vi "test_TCP_TCP Write.vi"(8 "error in (no error)":errorcluster, 11 "TestCase in":refnum<class "Ethernet Protocol Tests.lvclass">) -> (0 "error out":errorcluster, 3 "TestCase out":refnum<class "Ethernet Protocol Tests.lvclass">)   [LabVIEW 2019, in "Ethernet Protocol Tests.lvclass"]
uses:
  Ethernet Protocol Tests.lvclass
  ListenerVi/TCP/TCP.lvclass
  D:/GitRepository/niveristand-instrument-addon-classes/Source/Protocols/Tests/ListenerVi/Protocol Parent/Protocol Parent.lvclass
  ListenerVi/Listener.lvclass
  ListenerVi/ListenerClassControls/Operation Ctl.ctl
  ListenerVi/TCP/TCP.lvclass/TCP.ctl
  <vilib>/addons/_JKI Toolkits/VI Tester/TestCase.llb/TestCase.lvclass
  C:/Program Files (x86)/National Instruments/LabVIEW 2019/vi.lib/addons/_JKI Toolkits/VI Tester/TestCase.llb/TestCase.lvclass
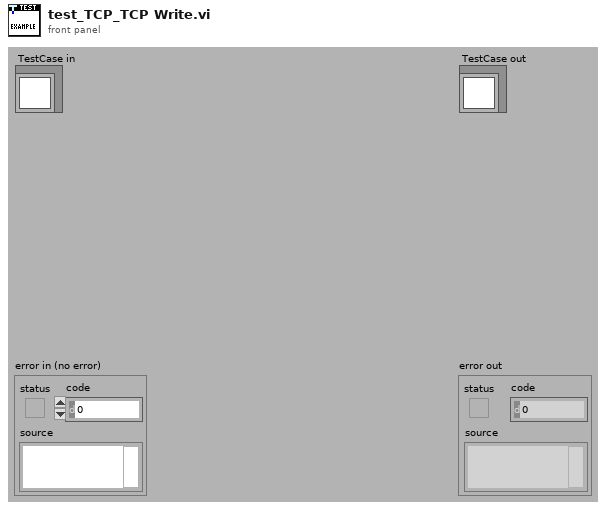
[diagram p1: front panel]
types:
  T1 = typedef "Operation Ctl.ctl" = enum16{"Read", "Write"}
  T2 = typedef "Listener.lvclass/TCP IP Data Structure.ctl" = cluster{"TCP|IP connection ID":refnum<k5>, "IP Address":string, "Port":u16, "Data":string}
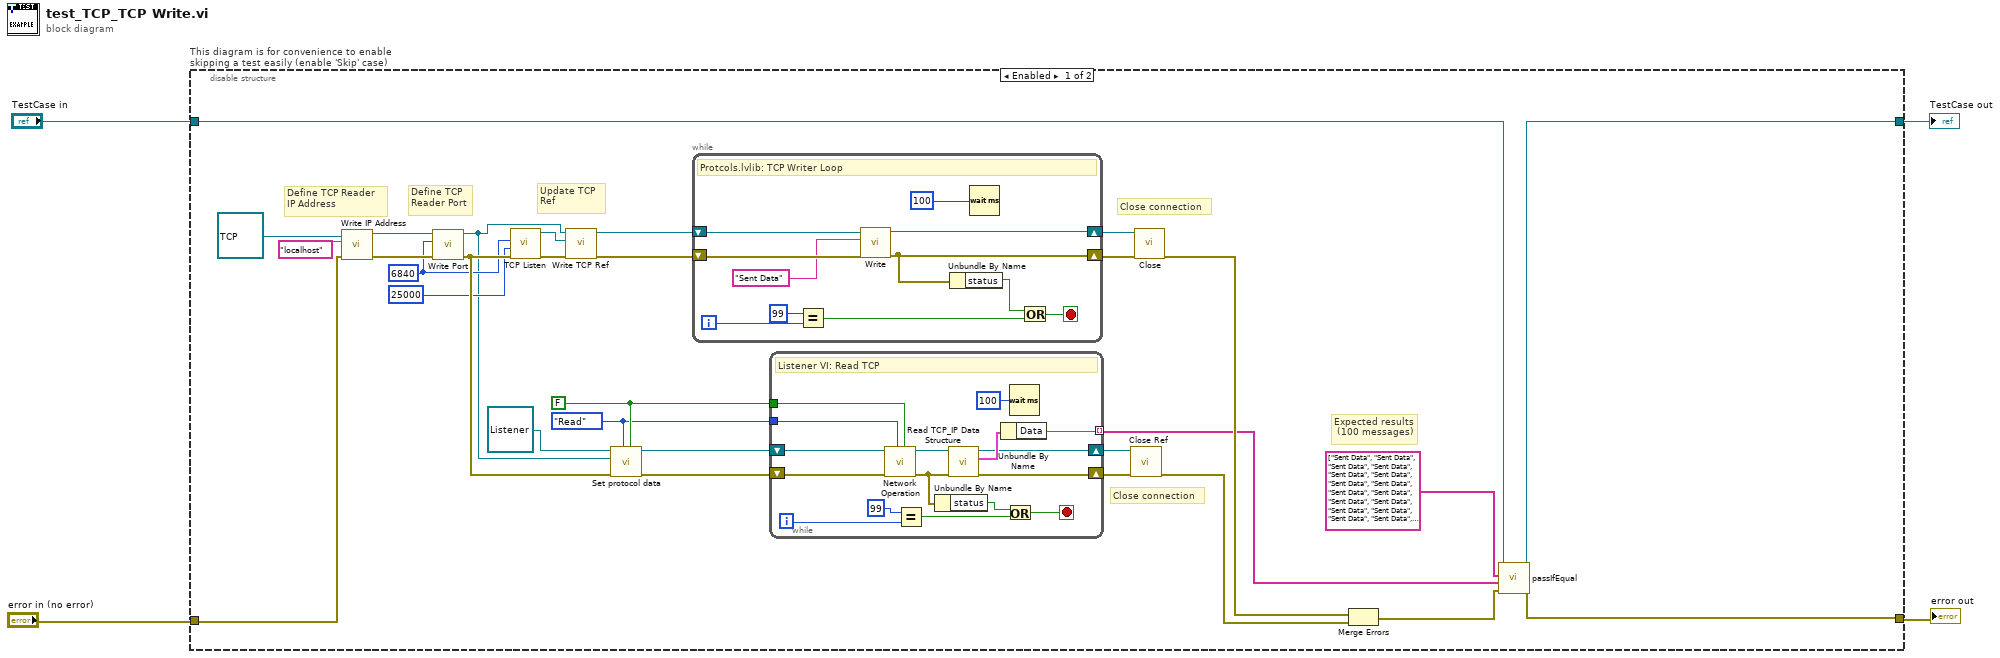
[diagram p0: block diagram]
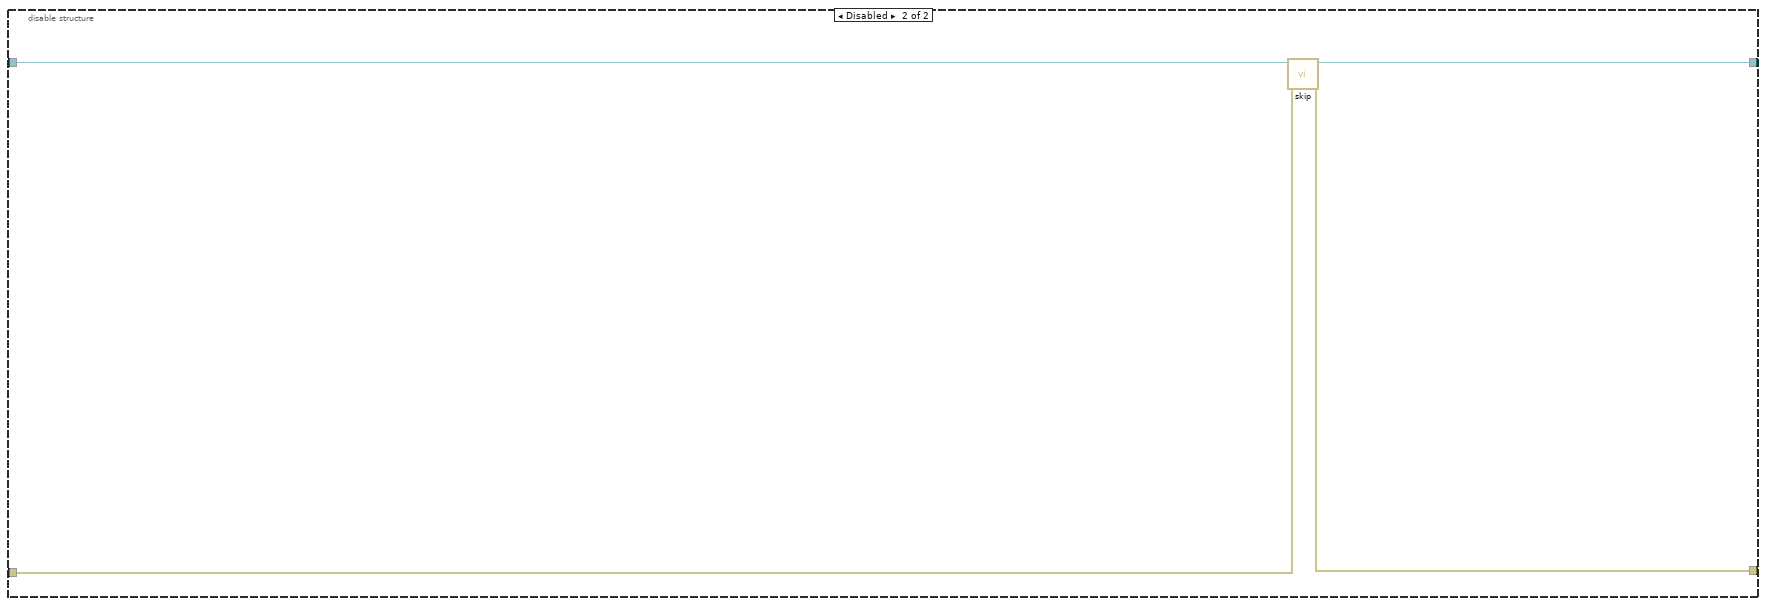
[diagram p2: hidden frame]
diagram:
  n1 = disable-structure "This diagram is for convenience to enable skipping a test easily (enable 'Skip' case)" shown="Enabled" {
    disable-tunnel: "TestCase in" -> [w34 w65]
    disable-tunnel: [w33 w63] -> w1
    disable-tunnel: [w32 w64] -> w3
    disable-tunnel: "error in (no error)" -> [w27 w62]
    frame Enabled {
      w13 = FALSE ("AK?")
      w12 = Operation_Ctl."Read" ("Operation")
      w20 = u16 6840 ("Port")
      # "Close connection"
      # "Close connection"
      # "Update TCP \nRef"
      # "Expected results\n (100 messages)"
      # "Define TCP \nReader Port"
      # "Define TCP Reader \nIP Address"
      n2 = call "Write IP Address.vi"("error in (no error)"=w27, "IP Address"="localhost", "Ethernet in"=refnum<class "TCP.lvclass"> refnum ("Localhost Protocols.lvlib:TCP.lvclass")) -> ("error out"=w28:errorcluster, "Ethernet out"=w29:refnum<class "TCP.lvclass">)  [unwired: 7 in]
      n3 = call "Write Port.vi"("error in (no error)"=w28, "Port"=w20, "Ethernet in"=w29) -> ("error out"=w21:errorcluster, "Ethernet out"=w15:refnum<class "TCP.lvclass">)  [unwired: 7 in]
      n4 = call <vilib>:"TCP Listen.vi"("error in (no error)"=w21, "timeout ms (wait forever: -1)"=25000, "port"=w20) -> ("error out"=w18:errorcluster, "connection ID"=w14:refnum<k5>)  [unwired: 4 in, 3 out]
      n5 = call "Write TCP Ref.vi"("error in (no error)"=w18, "TCP Ref"=w14, "Ethernet in"=w15) -> ("error out"=w17:errorcluster, "Ethernet out"=w16:refnum<class "TCP.lvclass">)  [unwired: 7 in]
      n6 = call "Set protocol data.vi"("AK?"=w13, "Operation"=w12, "error in (no error)"=w21, "Localhost Protocols.lvlib:Protocol Parent.lvclass"=w15, "Listener In.lvclass"=refnum<class "Listener.lvclass"> refnum ("Listener.lvclass")) -> ("error out"=w22:errorcluster, "Listener Out.lvclass"=w23:refnum<class "Listener.lvclass">)  [unwired: 5 in]
      n7 = while {
        shift-right: [w53] -> w8
        shift-left: w17 -> [w56]
        shift-right: [w52] -> w7
        shift-left: w16 -> [w55]
        i -> [w61]
        stop <- w58 stop-if-true
        # "Protcols.lvlib: TCP Writer Loop"
        n8 = Equal?(x=99, y=w61) -> (x = y?=w59:bool)
        n9 = call-dynamic "Write.vi"("error in (no error)"=w56, "String"="Sent Data", "Ethernet in"=w55) -> ("error out"=w53:errorcluster, "Ethernet out"=w52:refnum<class "TCP.lvclass">)  [unwired: 7 in]
        n10 = Unbundle By Name(w53) -> ("status"=w51:bool)
        n11 = Wait (ms)(milliseconds to wait=u32 100) -> ()  [unwired: 1 out]
        n12 = Or(x=w51, y=w59) -> (x .or. y?=w58:bool)
      }
      n13 = while {
        shift-right: [w36] -> w10
        shift-left: w22 -> [w50]
        shift-right: [w37] -> w11
        shift-left: w23 -> [w49]
        tunnel: w13 -> [w42]
        tunnel: w12 -> [w41]
        tunnel: [w35] -> w5 mode=indexing
        i -> [w46]
        stop <- w47 stop-if-true
        # "Listener VI: Read TCP"
        n14 = call "Network Operation.vi"("AK?"=w42, "Operation"=w41, "error in (no error)"=w50, "Listener In.lvclass"=w49) -> ("error out"=w40:errorcluster, "Listener Out.lvclass"=w39:refnum<class "Listener.lvclass">)  [unwired: 6 in]
        n15 = Equal?(x=99, y=w46) -> (x = y?=w44:bool)
        n16 = Unbundle By Name(w40) -> ("status"=w48:bool)
        n17 = call-dynamic "Read TCP_IP Data Structure.vi"("error in (no error)"=w40, "Listener in"=w39) -> ("error out"=w36:errorcluster, "TCP|IP Data Structure"=w38:T2, "Listener out"=w37:refnum<class "Listener.lvclass">)  [unwired: 7 in]
        n18 = Unbundle By Name(w38) -> ("Data"=w35:string)
        n19 = Or(x=w48, y=w44) -> (x .or. y?=w47:bool)
        n20 = Wait (ms)(milliseconds to wait=u32 100) -> ()  [unwired: 1 out]
      }
      n21 = call "Close Ref.vi"("error in (no error)"=w10, "Listener In.lvclass"=w11) -> ("error out"=w9:errorcluster)  [unwired: 9 in]
      n22 = call-dynamic "Close.vi"("error in (no error)"=w8, "Ethernet in"=w7) -> ("error out"=w6:errorcluster)  [unwired: 8 in, 1 out]
      n23 = Merge Errors(w6, w9) -> (w26:errorcluster)
      n24 = call-dynamic "passIfEqual.vi"("error in (no error)"=w26, "y"=w5, "x"=string[] ["Sent Data", "Sent Data", "Sent Data", "Sent Data", "Sent Data", "Sent Data", "Sent Data", "Sent Data", "Sent Data", "Sent Data", "Sent Data", "Sent Data", "Sent Data", "Sent Data", "Sent Data", "Sent Data", "Sent Data", "Sent Data", "Sent Data", "Sent Data", "Sent Data", "Sent Data", "Sent Data", "Sent Data", "Sent Data", "Sent Data", "Sent Data", "Sent Data", "Sent Data", "Sent Data", "Sent Data", "Sent Data", "Sent Data", "Sent Data", "Sent Data", "Sent Data", "Sent Data", "Sent Data", "Sent Data", "Sent Data", "Sent Data", "Sent Data", "Sent Data", "Sent Data", "Sent Data", "Sent Data", "Sent Data", "Sent Data", "Sent Data", "Sent Data", "Sent Data", "Sent Data", "Sent Data", "Sent Data", "Sent Data", "Sent Data", "Sent Data", "Sent Data", "Sent Data", "Sent Data", "Sent Data", "Sent Data", "Sent Data", "Sent Data", "Sent Data", "Sent Data", "Sent Data", "Sent Data", "Sent Data", "Sent Data", "Sent Data", "Sent Data", "Sent Data", "Sent Data", "Sent Data", "Sent Data", "Sent Data", "Sent Data", "Sent Data", "Sent Data", "Sent Data", "Sent Data", "Sent Data", "Sent Data", "Sent Data", "Sent Data", "Sent Data", "Sent Data", "Sent Data", "Sent Data", "Sent Data", "Sent Data", "Sent Data", "Sent Data", "Sent Data", "Sent Data", "Sent Data", "Sent Data", "Sent Data", "Sent Data"] ("Array"), "TestCase in"=w34) -> ("error out"=w32:errorcluster, "TestCase out"=w33:refnum<class "Ethernet Protocol Tests.lvclass">)  [unwired: 6 in]
    }
    frame Disabled {
      # "skip test result while test is under development"
      n25 = call <vilib>:"skip.vi"("error in (no error)"=w62, "TestCase in"=w65) -> ("error out"=w64:errorcluster, "TestCase out"=w63:refnum<class "Ethernet Protocol Tests.lvclass">)  [unwired: 8 in]
    }
  }
  "error out" <- w3
  "TestCase out" <- w1
